vi "Lidar 각도필터.vi"(3 "filter angle(plus)":dbl) -> (1 "거리 + 각도필터된 배열":dbl[][](array[numeric]))   [LabVIEW 2016]
panel:
  out "거리 + 각도필터된 배열 수":i32
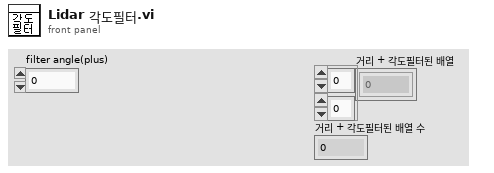
[diagram p1: front panel]
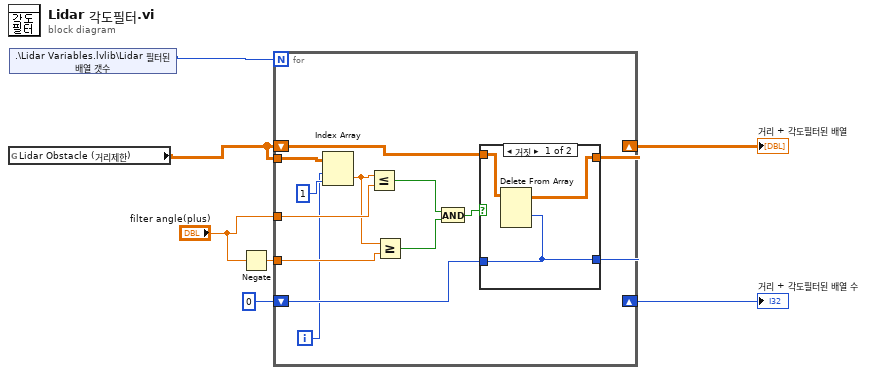
[diagram p0: block diagram]
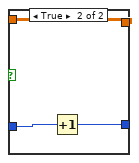
[diagram p2: hidden frame]
diagram:
  n1 = global read "[GV]_Lidar Obstacle (거리제한).vi" "Lidar Obstacle (거리제한)"() -> (w2:dbl[][])
  n2 = shared-variable ".\\Lidar Variables.lvlib\\Lidar 필터된 배열 갯수"() -> (w1:i32)  [unwired: 1 in, 1 out]
  n3 = Negate(x="filter angle(plus)") -> (-x=w6:dbl)
  n4 = for {
    N: w1 -> [_]
    tunnel: "filter angle(plus)" -> [w19]
    tunnel: w6 -> [w17]
    shift-right: [w10] -> w3
    shift-left: 0 ("비활성화된 인덱스 (행)") -> [w12]
    shift-right: [w11] -> w4
    shift-left: w2 -> [w13]
    tunnel: w2 -> [w9]
    i -> [w8]
    n5 = Index Array(array=w9, index (row)=w8, index (col)=1 ("비활성화된 인덱스 (열)")) -> (element=w18:dbl)
    n6 = Less Or Equal?(x=w18, y=w19) -> (x <= y?=w16:bool)
    n7 = Greater Or Equal?(x=w18, y=w17) -> (x >= y?=w15:bool)
    n8 = And(x=w16, y=w15) -> (x .and. y?=w14:bool)
    n9 = case shown="거짓" w14 {
      tunnel: w13 -> [w23 w24]
      tunnel: w12 -> [w21 w26]
      tunnel: [w22 w24] -> w11
      tunnel: [w21 w25] -> w10
      frame False {
        n10 = Delete From Array(array=w23, index (row)=w21) -> (array with subset deleted=w22:dbl[][])  [unwired: 2 in, 1 out]
      }
      frame True {
        n11 = Increment(x=w26) -> (x+1=w25:i32)
      }
    }
  }
  "거리 + 각도필터된 배열" <- w4
  "거리 + 각도필터된 배열 수" <- w3
